vi "Robot Global Data.vi"() -> ()   [LabVIEW 2020]
doc: "This global VI can contain as many global variables as you need. To create a global variable, place a control on the panel, give it a good name. To read or write to it from a VI, drag the icon to the diagram of that VI. You can also drag from the project. Click on the node to change which global you access. You shouldn't have multiple locations writing to a global or it will cause a race-condition."
uses:
  <vilib>/Rock Robotics/WPI/Camera/WPI_CameraImageSize.ctl
  <vilib>/Rock Robotics/WPI/DriverStation/WPI_DriverStationRobotMode2.ctl
panel:
  in  "Auto Pickup":string
  in  "Auto List":string
  in  "Spring Arm Setpoint":dbl
  in  "Climb Setpoint":dbl
  in  "Transfer Release Duration":dbl
  in  "Transfer Up Duration":dbl
  in  "Transfer Release Setpoint":dbl
  in  "Transfer Up Setpoint":dbl
  in  "Record Path":bool
  in  "Wheel":dbl
  in  "Throtle":dbl
  in  "Op Button 11":bool
  in  "Op Button 10":bool
  in  "Op Button 9":bool
  in  "Op Button 8":bool
  in  "Spring Arm":bool
  in  "Button 11":bool
  in  "Button 10":bool
  in  "Button 9":bool
  in  "Button 8":bool
  in  "Button 7":bool
  in  "Button 6":bool
  in  "Button 5":bool
  in  "Button 4":bool
  in  "Record Path Stop RB":bool
  in  "Record Path Start LB":bool
  in  "Pivot Right RT":bool
  in  "Pivot Left LT":bool
  in  "Climb Traversal":bool
  in  "Transfer Release":bool
  in  "Transfer Up":bool
  in  "Intake Arm Down LT":bool
  in  "Intake Arm Up LB":bool
  in  "Intake RT":bool
  in  "Shooter RB":bool
  in  "Intake Setpoint":dbl=0.8 format="%#_13g"
  in  "Intake Duration (s)":dbl=3.0 format="%#_13g"
  in  "Shooter Duration (s)":dbl=3.0 format="%#_13g"
  in  "Shooter Setpoint":dbl=0.8 format="%#_13g"
  in  "Robot Mode":T1
  in  "image size":T2=enum."320x240"
  in  "Enable Vision":bool
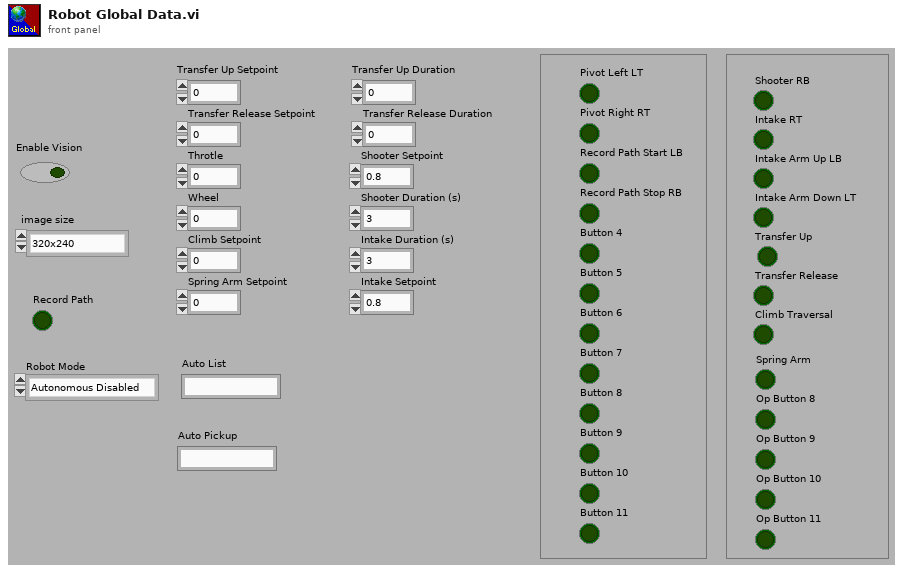
[diagram p1: front panel]
types:
  T1 = typedef "WPI_DriverStationRobotMode2.ctl" = enum16{"Autonomous Disabled", "Autonomous Enabled", "Teleop Disabled", "Teleop Enabled", "Disconnected", "Finish", "Test Disabled", "Test Enabled", "Emergency Stopped"}
  T2 = typedef "WPI_CameraImageSize.ctl" = enum16{"640x480", "320x240", "160x120", "Custom"}
diagram:
